vi "VFH-read_file-LabVIEW.vi"(8 "error in":errorcluster, 10 "file path (dialog if empty)":path=path "C:/projects/UNI/VNA/MiniVNA/20240625-162312-Vann/Vann.txt") -> (0 "error out":errorcluster, 2 "output cluster":T1)   [LabVIEW 2020, in "VFH-VNA_File_Handler.lvlib"]
uses:
  VFH-VNA_File_Handler.lvlib
  VFH-file_cluster-LabVIEWVNA.ctl
panel:
  out "string array 2":string[][](array[string])
  out "string array":string[](array[string])
  out "after substring":string
  out "text":string
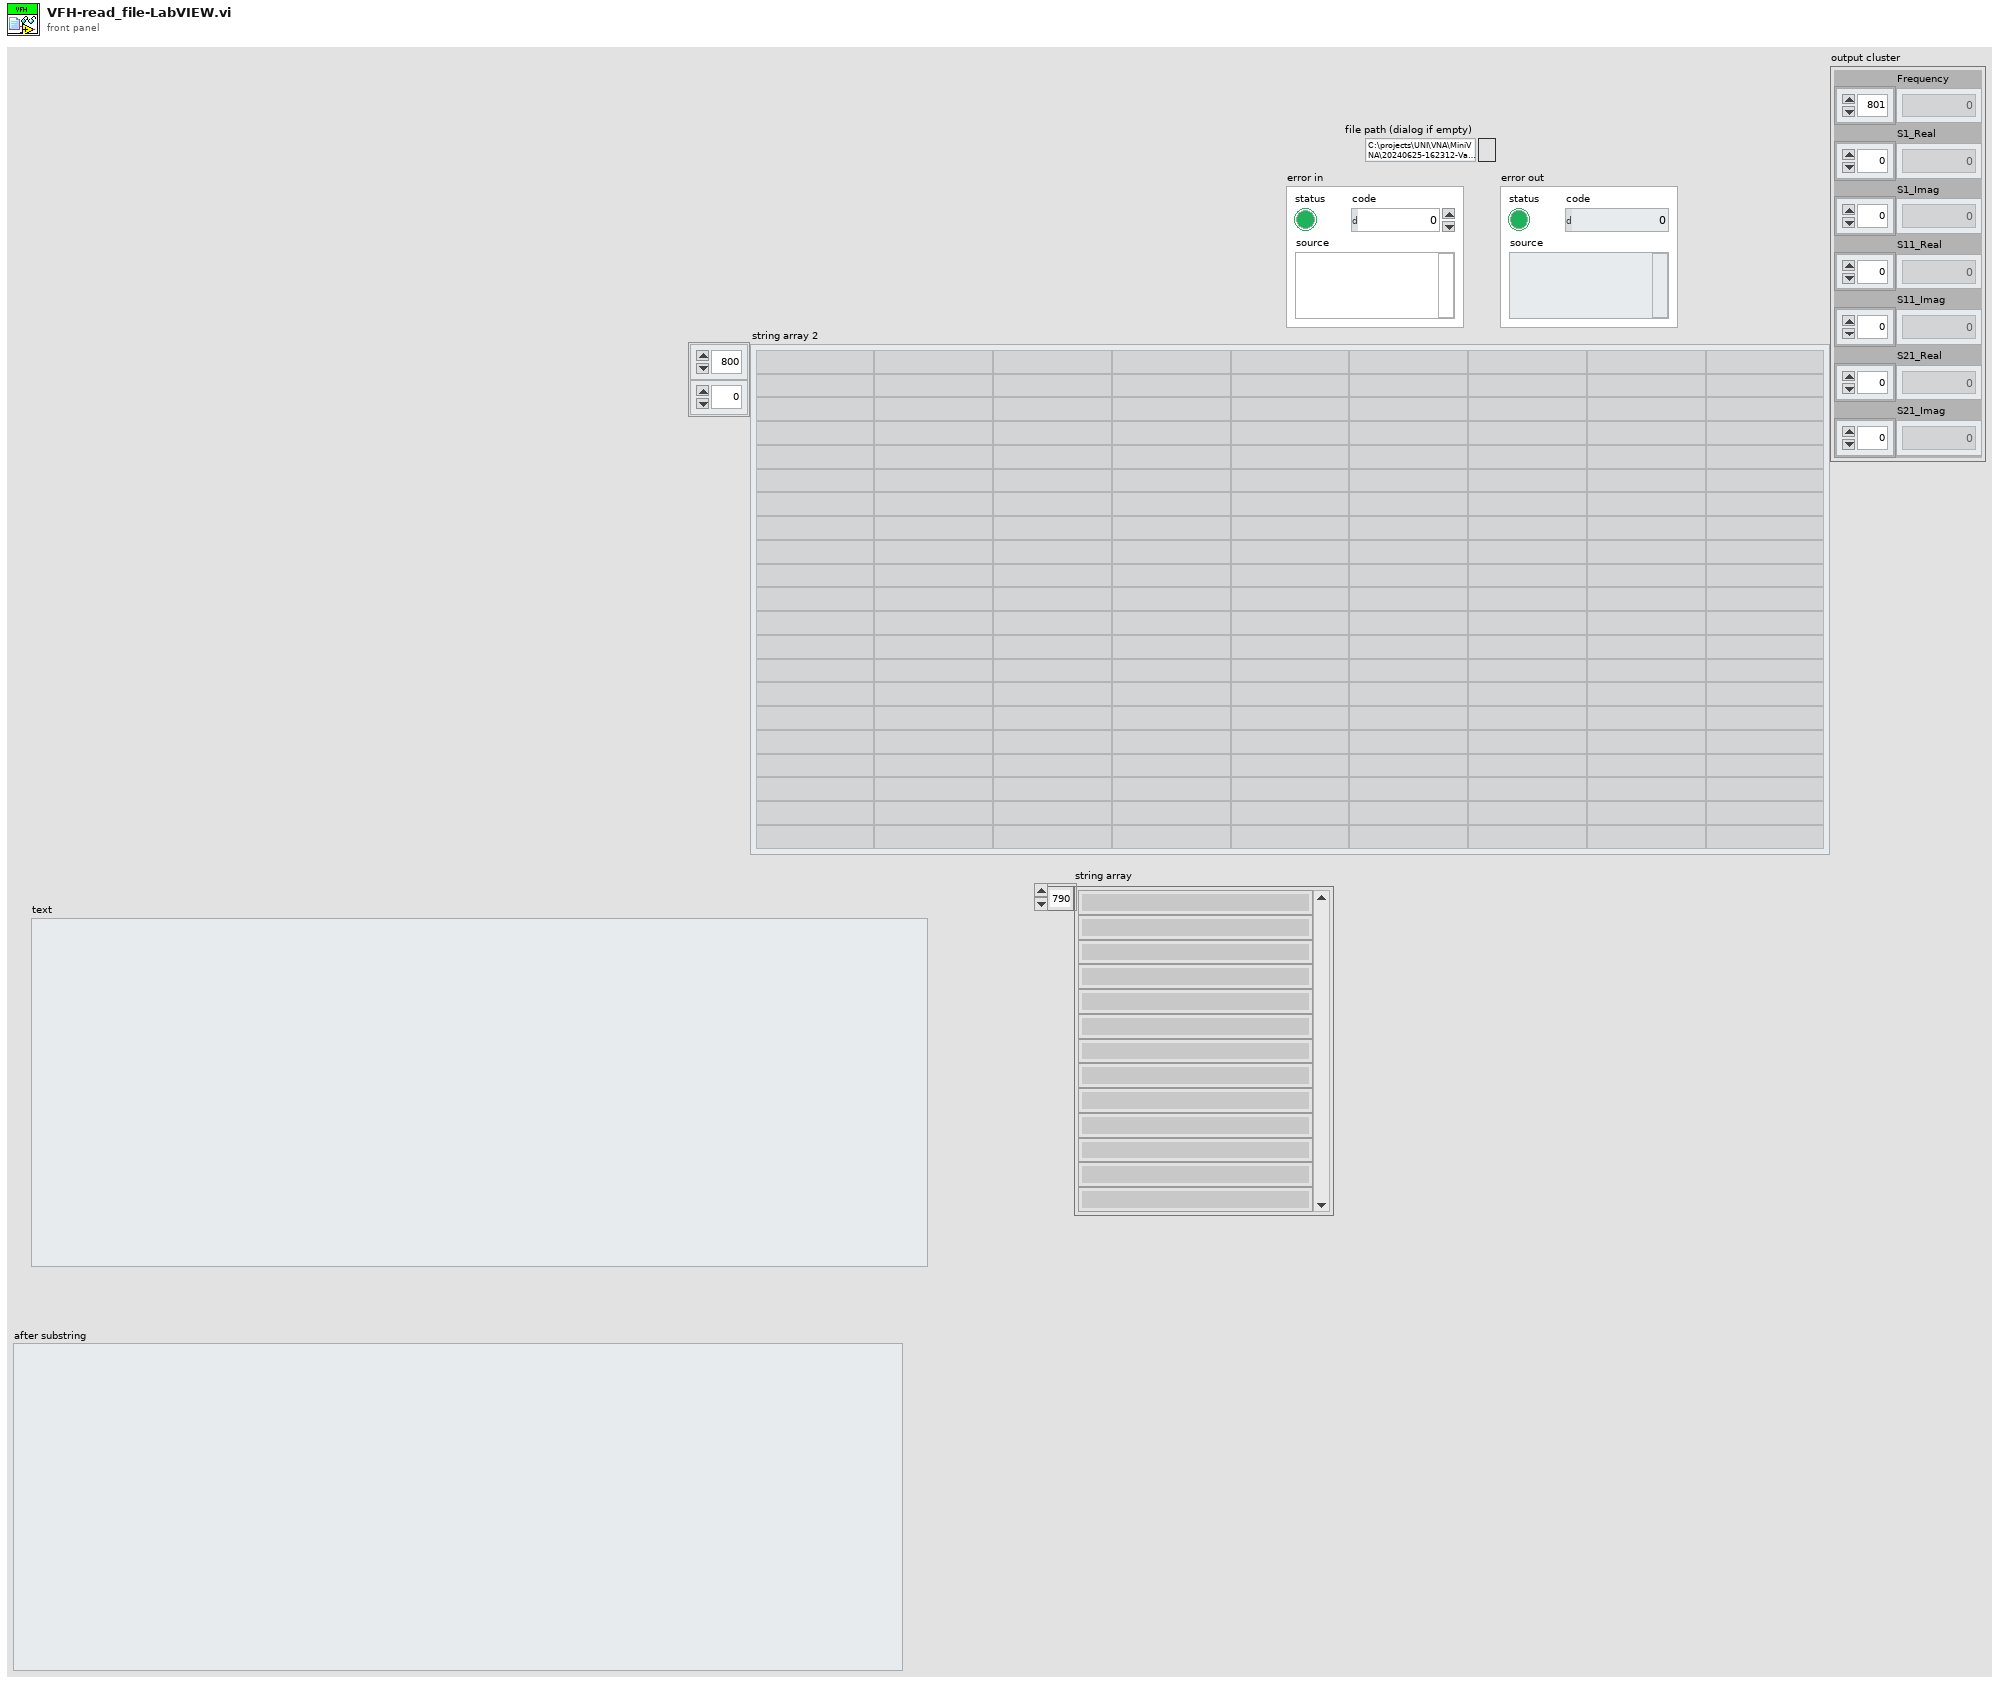
[diagram p1: front panel]
types:
  T1 = typedef "VFH-VNA_File_Handler.lvlib/VFH-file_cluster-LabVIEWVNA.ctl" = cluster{"Frequency":dbl[], "S1_Real":dbl[], "S1_Imag":dbl[], "S11_Real":dbl[], "S11_Imag":dbl[], "S21_Real":dbl[], "S21_Imag":dbl[]}
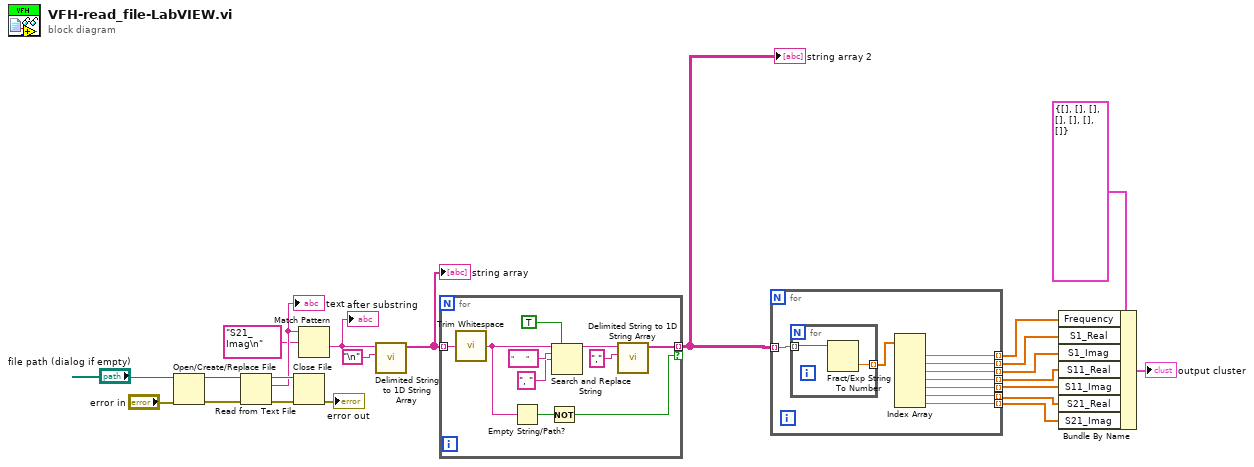
[diagram p0: block diagram]
diagram:
  n1 = Open/Create/Replace File(file path (use dialog)="file path (dialog if empty)", error in="error in") -> (refnum out=w22:refnum<file>, error out=w19:errorcluster)  [unwired: 4 in, 1 out]
  n2 = Read from Text File(file (use dialog)=w22, error in=w19) -> (refnum out=w21:refnum<file>, text=w17:string, error out=w20:errorcluster)  [unwired: 2 in, 1 out]
  "text" <- w17
  n3 = Close File(refnum=w21, error in=w20) -> (error out=→"error out":errorcluster)  [unwired: 1 out]
  n4 = Match Pattern(string=w17, regular expression="S21_Imag\n" ("search string/char (-)")) -> (after substring=w13:string)  [unwired: 1 in, 3 out]
  "after substring" <- w13
  n5 = call <vilib>:"Delimited String to 1D String Array.vi"("delimiter"="\n", "delimited string"=w13) -> ("string array"=w14:string[])  [unwired: 9 in]
  "string array" <- w14
  n6 = for {
    tunnel: w14 -> [w32] mode=indexing
    tunnel: [w31] -> w12 mode=indexing if=w23
    n7 = call <vilib>:"Trim Whitespace.vi"("string"=w32) -> ("trimmed string"=w25:string)  [unwired: 1 in]
    n8 = Empty String/Path?(string/path=w25) -> (empty?=w24:bool)
    n9 = Not(x=w24) -> (.not. x?=w23:bool)
    n10 = Search and Replace String(replace all?=TRUE ("replace all? (F)"), input string=w25, search string="      ", replace string=", " ("replace string (\"\")")) -> (result string=w26:string)  [unwired: 4 in, 3 out]
    n11 = call <vilib>:"Delimited String to 1D String Array.vi"("delimiter"=",", "delimited string"=w26) -> ("string array"=w31:string[])  [unwired: 9 in]
  }
  "string array 2" <- w12
  n12 = for {
    tunnel: w12 -> [w41] mode=indexing
    tunnel: [w39] -> w11 mode=indexing
    tunnel: [w38] -> w10 mode=indexing
    tunnel: [w37] -> w9 mode=indexing
    tunnel: [w36] -> w8 mode=indexing
    tunnel: [w35] -> w7 mode=indexing
    tunnel: [w34] -> w6 mode=indexing
    tunnel: [w33] -> w5 mode=indexing
    n13 = for {
      tunnel: w41 -> [w43] mode=indexing
      tunnel: [w42] -> w40 mode=indexing
      n14 = Fract/Exp String To Number(string=w43) -> (number=w42:dbl)  [unwired: 3 in, 1 out]
    }
    n15 = Index Array(array=w40) -> (element #1=w39:dbl, element #2=w38:dbl, element #3=w37:dbl, element #4=w36:dbl, element #5=w35:dbl, element #6=w34:dbl, element #7=w33:dbl)  [unwired: 7 in]
  }
  n16 = Bundle By Name(cluster=T1 {"Frequency"=[], "S1_Real"=[], "S1_Imag"=[], "S11_Real"=[], "S11_Imag"=[], "S21_Real"=[], "S21_Imag"=[]} ("output cluster"), "Frequency"=w11, "S1_Real"=w10, "S1_Imag"=w9, "S11_Real"=w8, "S11_Imag"=w7, "S21_Real"=w6, "S21_Imag"=w5) -> (→"output cluster":T1)
